vi "Bang Bang Temperature Controller.vi"() -> ()   [LabVIEW 2021]
uses:
  Source/Support/Nodes/Decorators/Repeater/Support/Finish On - Type.ctl
  <vilib>/TSA/Omni-Bus/Omni-Bus/Omni_Bus.lvclass
  <vilib>/TSA/Omni-Bus/Local Bus/Support/Tag List Type.ctl
  <vilib>/Utility/Data Type/Type Definitions/Data Type.ctl
  <vilib>/TSA/Omni-Bus/Local Bus/Local Bus.lvclass
  C:/Program Files (x86)/National Instruments/LabVIEW 2021/vi.lib/TSA/Omni-Bus/Omni-Bus/Bus Access/Bus_Access.lvclass
  Test System/Test System.lvclass
  C:/Users/Tim/Documents/GitHub/LV_Behaviour_Tree/Source/Support/abs_System/bt_System.lvclass
  Source/Support/Nodes/abs_Node/Status.ctl
  Test System/Test System.lvclass/Test System.ctl
  <vilib>/TSA/Omni-Bus/Omni-Bus/Support/Get/Static/Get Static Boolean.vi
  <vilib>/TSA/Omni-Bus/Omni-Bus/Support/Get/Static/Get Static DBL.vi
  <vilib>/TSA/Omni-Bus/Omni-Bus/Support/Write/Write DBL.vi
  <vilib>/TSA/Omni-Bus/Omni-Bus/Support/Read/Read Boolean.vi
  Test System/Properties/Read Log Messages.vi
  <vilib>/TSA/Abstract Data Classes/Constants/Support/DBL/Const_DBL.lvclass
  C:/Program Files (x86)/National Instruments/LabVIEW 2021/vi.lib/TSA/Abstract Data Classes/Abs_Types/Double Float/Abs_Double Float.lvclass
  <vilib>/TSA/Abstract Data Classes/Constants/Support/DBL/DBL.vi
  <vilib>/TSA/Abstract Data Classes/Abs_Types/Double Float/Abs_Double Float.lvclass
  <vilib>/TSA/Abstract Data Classes/Abs_Types/Boolean/Abs_Boolean.lvclass
  Source/Support/Nodes/abs_Node/bt_Node.lvclass
  Source/BT.lvlib
  Source/Support/Nodes/Decorators/Repeater/bt_Repeater.lvclass
  <vilib>/Utility/Data Type/NI_Data Type.lvlib
panel:
  out "Waveform Chart":cluster{"Temperature Reading":dbl, i16}(graph)
  in  "stop":bool
  in  "Temperature Reading":dbl(slide) scale=0.0..100.0
  out "Heater":bool
  in  "Hystersis":dbl=2.0
  in  "Temperature Setting":dbl=50.0
  out "Log Messages":string[](array[string])
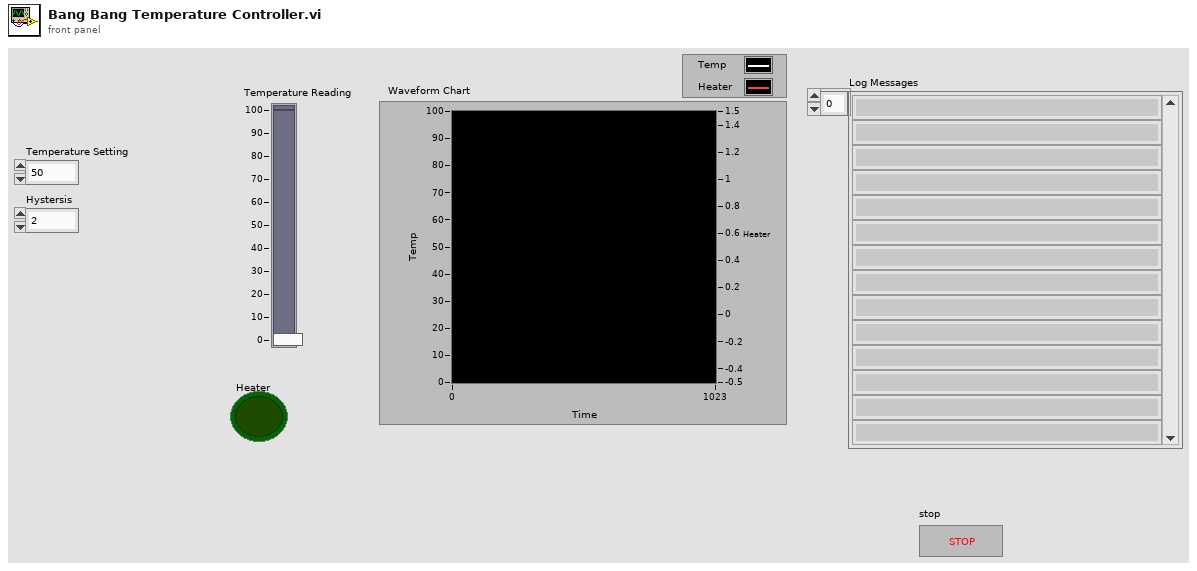
[diagram p1: front panel]
types:
  T1 = typedef "Local Bus.lvclass/Tag List Type.ctl" = cluster{"Tag":string, "Type":T2}
  T2 = typedef "NI_Data Type.lvlib/Data Type.ctl" = enum8{"Invalid Type", "Void", "I8", "I16", "I32", "I64", "U8", "U16", "U32", "U64", "Single Float", "Double Float", "Extended Float", "Single Complex", "Double Complex", "Extended Complex", "Enum U8", "Enum U16", "Enum U32", "Enum U64", "Single Float With Unit", "Double Float With Unit", "Extended Float With Unit", "Single Complex with Unit", "Double Complex with Unit", "Extended Complex with Unit", "Boolean", "String", "Path", "Picture", "Tag", "Array", "Cluster", "Variant", "LV Variant", "Waveform", "Timestamp", "Digital Waveform", "Digital Data", "ExpressData", "Refnum", "External Data", "VI", "Poly VI", "LabVIEW Class Instance", "Fixed Point", "Set Collection", "Map Collection"}
  T3 = typedef "BT.lvlib/bt_Repeater.lvclass/Finish On - Type.ctl" = enum16{"Success", "Failure", "Never"}
  T4 = typedef "BT.lvlib/bt_Node.lvclass/Status.ctl" = enum16{"Success", "Failure", "Running"}
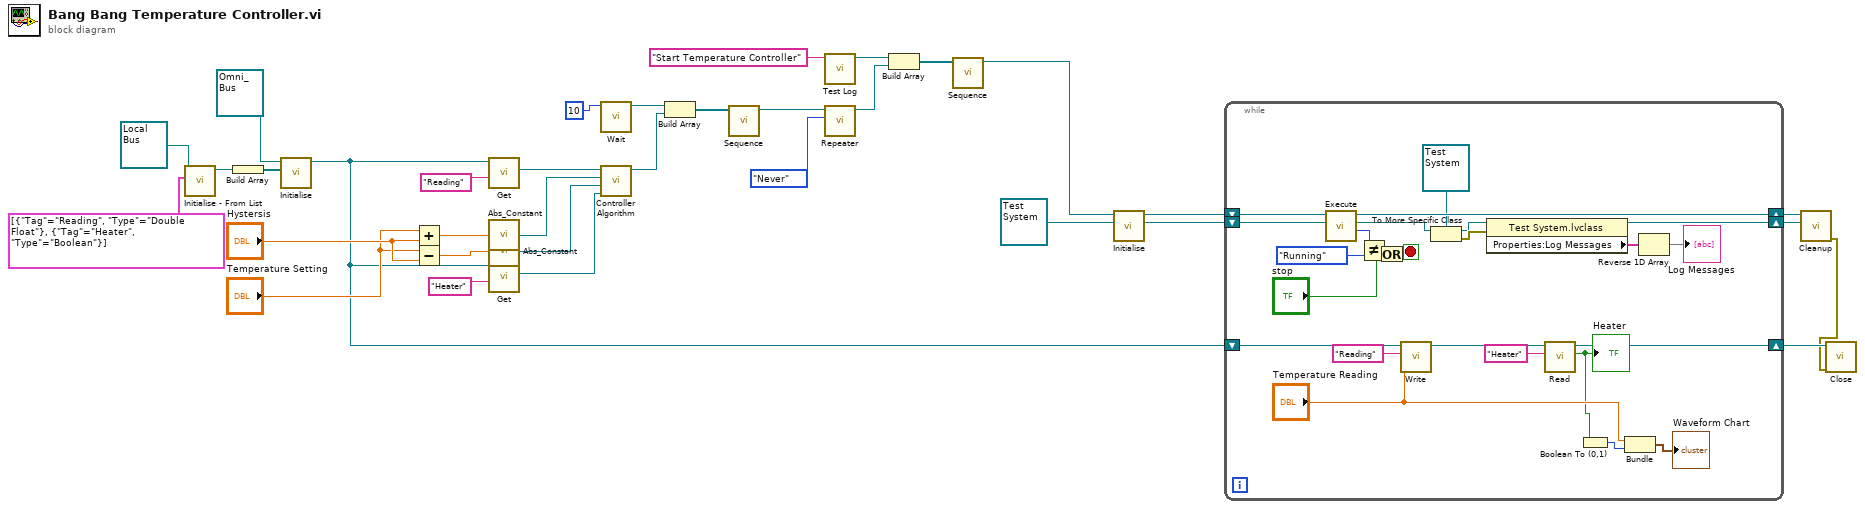
[diagram p0: block diagram]
diagram:
  n1 = call <vilib>:"Initialise - From List.vi"("Tag List"=T1[] [{"Tag"="Reading", "Type"=enum."Double Float"}, {"Tag"="Heater", "Type"=enum."Boolean"}], "Local Bus in"=refnum<class "Local Bus.lvclass"> refnum) -> ("Local Bus out"=w11:refnum<class "Local Bus.lvclass">)  [unwired: 8 in, 1 out]
  n2 = Build Array(w11) -> (w12:refnum<class "Local Bus.lvclass">[])
  n3 = call-dynamic "Initialise.vi"("Bus Access"=w12, "Var Bus in"=refnum<class "Omni_Bus.lvclass"> refnum) -> ("Var Bus out"=w9:refnum<class "Omni_Bus.lvclass">)  [unwired: 8 in, 1 out]
  n4 = Add(x="Temperature Setting", y="Hystersis") -> (x+y=w22:dbl)
  n5 = Subtract(x="Temperature Setting", y="Hystersis") -> (x-y=w21:dbl)
  n6 = call-poly <vilib>:"Get.vi"("Tag"="Reading", "Var Bus in"=w9) -> ("Value Out"=w28:refnum<class "Abs_Double Float.lvclass">)  [unwired: 7 in, 2 out]
  n7 = call-poly <vilib>:"Abs_Constant.vi"("Value"=w22) -> ("Constant"=w27:refnum<class "Const_DBL.lvclass">)  [unwired: 4 in]
  n8 = call-poly <vilib>:"Abs_Constant.vi"("Value"=w21) -> ("Constant"=w26:refnum<class "Const_DBL.lvclass">)  [unwired: 4 in]
  n9 = call-poly <vilib>:"Get.vi"("Tag"="Heater", "Var Bus in"=w9) -> ("Value Out"=w25:refnum<class "Abs_Boolean.lvclass">)  [unwired: 7 in, 2 out]
  n10 = call "Wait.vi"("Time (ms)"=u32 10) -> ("Node Out"=w16:refnum<class "bt_Node.lvclass">)  [unwired: 10 in]
  n11 = call "Controller Algorithm.vi"("Heater Output"=w25, "Lower Limit"=w26, "Upper Limit"=w27, "Reading"=w28) -> ("Node Out"=w18:refnum<class "bt_Node.lvclass">)  [unwired: 7 in]
  n12 = Build Array(w16, w18) -> (w17:refnum<class "bt_Node.lvclass">[])
  n13 = call "Sequence.vi"("Nodes"=w17) -> ("Node"=w14:refnum<class "bt_Node.lvclass">)  [unwired: 10 in]
  n14 = call "Test Log.vi"("Message"="Start Temperature Controller") -> ("BT.lvlib:abs_Node.lvclass"=w1:refnum<class "bt_Node.lvclass">)  [unwired: 10 in]
  n15 = call "Repeater.vi"("Finish On"=Finish_On_-_Type."Never", "Node In"=w14) -> ("Node Out"=w4:refnum<class "bt_Node.lvclass">)  [unwired: 9 in]
  n16 = Build Array(w1, w4) -> (w5:refnum<class "bt_Node.lvclass">[])
  n17 = call "Sequence.vi"("Nodes"=w5) -> ("Node"=w3:refnum<class "bt_Node.lvclass">)  [unwired: 10 in]
  n18 = call-dynamic "Initialise.vi"("System In"=refnum<class "Test System.lvclass"> refnum ("Test System.lvclass"), "Node in"=w3) -> ("System Out"=w32:refnum<class "bt_System.lvclass">, "Node out"=w33:refnum<class "bt_Node.lvclass">)  [unwired: 7 in, 1 out]
  n19 = while {
    shift-right: [w56] -> w31
    shift-left: w33 -> [w58]
    shift-right: [w52] -> w30
    shift-left: w32 -> [w57]
    shift-right: [w43] -> w7
    shift-left: w9 -> [w45]
    stop <- w40 stop-if-true
    n20 = call-dynamic "Execute.vi"("System In"=w57, "Node in"=w58) -> ("Status"=w55:T4, "System Out"=w50:refnum<class "bt_System.lvclass">, "Node out"=w56:refnum<class "bt_Node.lvclass">)  [unwired: 6 in, 1 out]
    n21 = Not Equal?(x=w55, y=Status."Running") -> (x != y?=w53:bool)
    n22 = Or(x=w53, y="stop") -> (x .or. y?=w40:bool)
    n23 = call-poly <vilib>:"Write.vi"("Numeric"="Temperature Reading", "Tag"="Reading", "Omni_Bus in"=w45) -> ("Omni_Bus out"=w44:refnum<class "Omni_Bus.lvclass">)  [unwired: 7 in, 1 out]
    n24 = To More Specific Class(target class=refnum<class "Test System.lvclass"> refnum ("Test System.lvclass"), reference=w50) -> (specific class reference=w49:refnum<class "Test System.lvclass">, error out=w51:errorcluster)  [unwired: 1 in]
    n25 = property class="Test System.lvclass"(reference=w49, error in=w51) -> (reference out=w52:refnum<class "Test System.lvclass">, "Properties:Log Messages"=w47:string[])  [unwired: 1 out]
    n26 = call-poly <vilib>:"Read.vi"("Tag"="Heater", "Var Bus in"=w44) -> ("Boolean"=w36:bool, "Var Bus out"=w43:refnum<class "Omni_Bus.lvclass">)  [unwired: 7 in, 1 out]
    "Heater" <- w36
    n27 = Boolean To (0,1)(Boolean=w36) -> (0, 1=w37:i16)
    n28 = Bundle("Temperature Reading"="Temperature Reading", w37) -> (→"Waveform Chart":cluster{"Temperature Reading":dbl, i16})  [unwired: 1 in]
    n29 = Reverse 1D Array(array=w47) -> (reversed array=→"Log Messages":string[])
  }
  n30 = call-dynamic "Cleanup.vi"("System In"=w30, "Node in"=w31) -> ("error out"=w6:errorcluster)  [unwired: 7 in, 2 out]
  n31 = call-dynamic "Close.vi"("error in (no error)"=w6, "Data in"=w7) -> ()  [unwired: 8 in, 2 out]
